vi "Get Parameter Definition Element Names.vi"() -> (3 "names":T1)   [LabVIEW 2020, in "AIM MIL-STD-1553 System Explorer.lvlib" / "Implementation.lvlib" / "Refresh.lvlib"]
uses:
  Refresh.lvlib
  Scripting/Constants.vi
  Scripting/AIM MIL-STD-1553 Scripting.lvlib
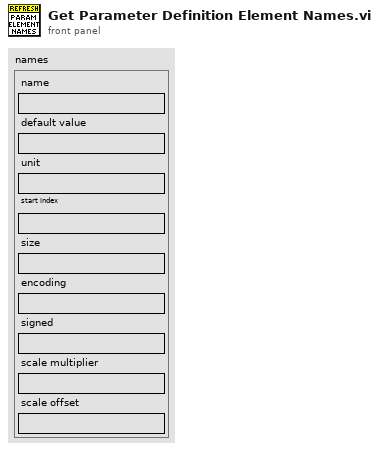
[diagram p1: front panel]
types:
  T1 = cluster{"name":string, "default value":string, "unit":string, "start index":string, "size":string, "encoding":string, "signed":string, "scale multiplier":string, "scale offset":string}
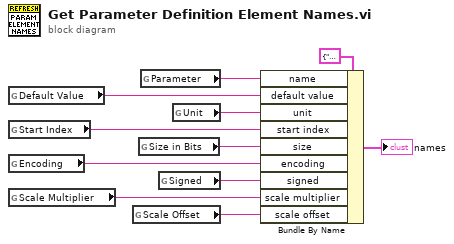
[diagram p0: block diagram]
diagram:
  n1 = global read "Constants.vi" "Default Value"() -> (w9:string)
  n2 = global read "Constants.vi" "Start Index"() -> (w7:string)
  n3 = global read "Constants.vi" "Encoding"() -> (w5:string)
  n4 = global read "Constants.vi" "Scale Multiplier"() -> (w3:string)
  n5 = global read "Constants.vi" "Scale Offset"() -> (w2:string)
  n6 = global read "Constants.vi" "Size in Bits"() -> (w6:string)
  n7 = global read "Constants.vi" "Parameter"() -> (w10:string)
  n8 = global read "Constants.vi" "Signed"() -> (w4:string)
  n9 = global read "Constants.vi" "Unit"() -> (w8:string)
  n10 = Bundle By Name(cluster=T1 {"name"="", "default value"="", "unit"="", "start index"="", "size"="", "encoding"="", "signed"="", "scale multiplier"="", "scale offset"=""} ("name strings"), "name"=w10, "default value"=w9, "unit"=w8, "start index"=w7, "size"=w6, "encoding"=w5, "signed"=w4, "scale multiplier"=w3, "scale offset"=w2) -> (→"names":T1)
